vi "HAL_Tester.vi"() -> ()   [LabVIEW 2024]
doc: "HAL Example utilizing classes and interfaces\n--------\nPaulo Rossi\nprossi@aurumautomation.ca\n©2024 Aurum Automation Inc.\nOpen-Sourced per GNU GPL v3\n\nYou should have received a copy of the GNU General Public License along with this program. If not, see <https://www.gnu.org/licenses/>."
uses:
  Keysight_PSU/Keithley_PSU.lvclass
  NI_PSU/NI_PSU.lvclass
  DAQ/DAQ.lvclass
  DMM/DMM_Concrete.lvclass
  Switch_Concrete/Switch_Concrete.lvclass
  PSU/PSU.lvclass
  SWITCH/SWITCH.lvclass
  DMM/DMM.lvclass
panel:
  in  "Switch Selector":bool
  in  "DMM Selector":bool
  out "Measured Voltage (V)":dbl
  in  "PSU Selector":bool
  out "error out":errorcluster
  in  "error in (no error)":errorcluster
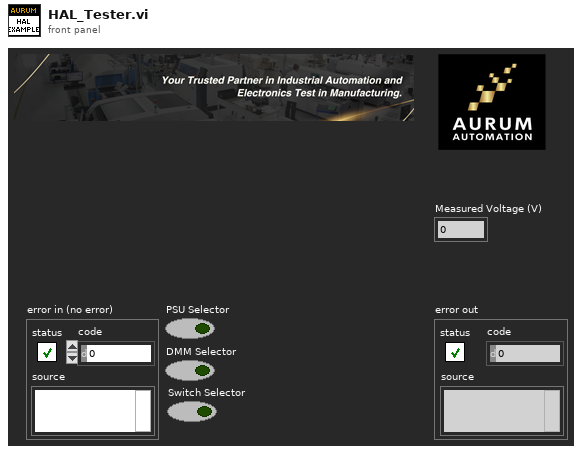
[diagram p1: front panel]
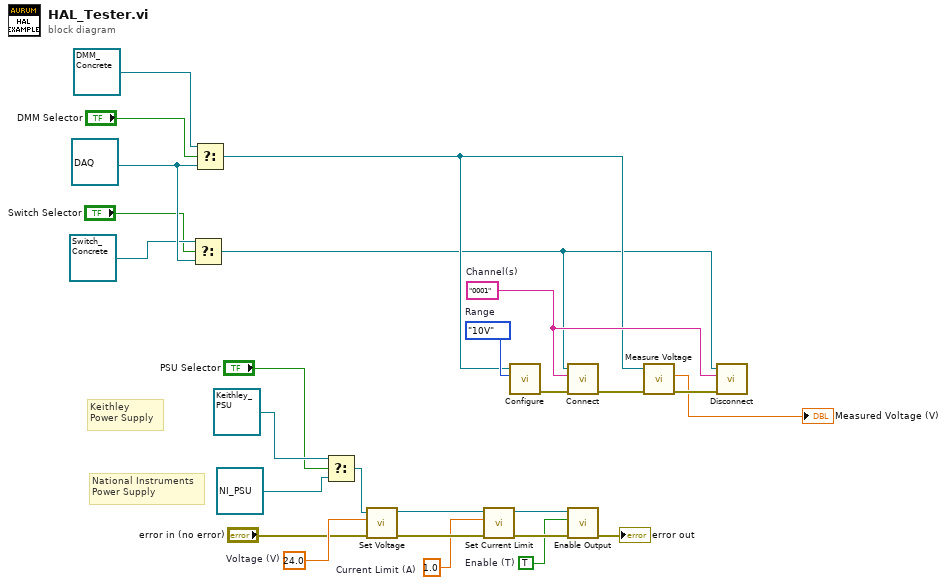
[diagram p0: block diagram]
diagram:
  w10 = "0001"  # Channel(s)
  w11 = enum16{"1V", "10V", "100V"}."10V"  # Range
  w8 = refnum<class "DAQ.lvclass"> refnum ("HAL.lvlib:DAQ.lvclass")
  w17 = TRUE  # Enable (T)
  w18 = 1.0  # Current Limit (A)
  w19 = 24.0  # Voltage (V)
  # "National Instruments\nPower Supply"
  # "Keithley\nPower Supply"
  n1 = Select(t=refnum<class "Switch_Concrete.lvclass"> refnum ("HAL.lvlib:Switch_Concrete.lvclass"), s="Switch Selector", f=w8) -> (s? t:f=w4:refnum<class "SWITCH.lvclass">)
  n2 = Select(t=refnum<class "DMM_Concrete.lvclass"> refnum ("HAL.lvlib:DMM_Concrete.lvclass"), s="DMM Selector", f=w8) -> (s? t:f=w5:refnum<class "DMM.lvclass">)
  n3 = Select(t=refnum<class "Keithley_PSU.lvclass"> refnum ("HAL.lvlib:Keysight_PSU.lvclass"), s="PSU Selector", f=refnum<class "NI_PSU.lvclass"> refnum ("HAL.lvlib:NI_PSU.lvclass")) -> (s? t:f=w24:refnum<class "PSU.lvclass">)
  n4 = call-dynamic "Set Voltage.vi"("error in (no error)"="error in (no error)", "Voltage (V)"=w19, "PSU in"=w24) -> ("error out"=w20:errorcluster, "PSU out"=w23:refnum<class "PSU.lvclass">)  [unwired: 7 in]
  n5 = call-dynamic "Set Current Limit.vi"("error in (no error)"=w20, "Current Limit (A)"=w18, "PSU in"=w23) -> ("error out"=w21:errorcluster, "PSU out"=w22:refnum<class "PSU.lvclass">)  [unwired: 7 in]
  n6 = call-dynamic "Configure.vi"("Range"=w11, "DMM in"=w5) -> ("error out"=w14:errorcluster)  [unwired: 8 in, 1 out]
  n7 = call-dynamic "Connect.vi"("error in (no error)"=w14, "Channel(s)"=w10, "SWITCH in"=w4) -> ("error out"=w13:errorcluster)  [unwired: 7 in, 1 out]
  n8 = call-dynamic "Enable Output.vi"("error in (no error)"=w21, "Enable (T)"=w17, "PSU in"=w22) -> ("error out"=→"error out":errorcluster)  [unwired: 7 in, 1 out]
  n9 = call-dynamic "Measure Voltage.vi"("error in (no error)"=w13, "DMM in"=w5) -> ("error out"=w12:errorcluster, "Voltage (V)"=→"Measured Voltage (V)":dbl)  [unwired: 7 in, 1 out]
  n10 = call-dynamic "Disconnect.vi"("error in (no error)"=w12, "Channel(s)"=w10, "SWITCH in"=w4) -> ()  [unwired: 7 in, 2 out]
